vi "Read Joystick.vi"(8 "Joystick Deadbanded Value (default of 0.1)":dbl, 11 "Joystick L 1 DevRef":T1) -> (1 "Joystick L 2 X Axis":dbl, 2 "Joystick L 1 Y Axis":dbl, 3 "Joystick L 1 X Axis":dbl)   [LabVIEW 2014]
uses:
  <vilib>/Rock Robotics/WPI/Joystick/WPI_JoystickDevRef.ctl
  <vilib>/Rock Robotics/WPI/Joystick/WPI_JoystickDeviceEnum.ctl
  Global Variables.vi
  <vilib>/Rock Robotics/WPI/Joystick/WPI_JoystickGetSetRefNum.vi
  <vilib>/Utility/file.llb/Write To Spreadsheet File (DBL).vi
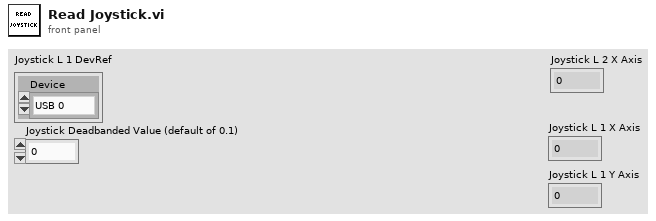
[diagram p1: front panel]
types:
  T1 = typedef "WPI_JoystickDevRef.ctl" = cluster{"Device":T2}
  T2 = typedef "WPI_JoystickDeviceEnum.ctl" = enum16{"USB 0", "USB 1", "USB 2", "USB 3", "USB 4", "USB 5"}
  T3 = cluster{"Buttons[0]":bool, "Buttons[1]":bool, "Buttons[2]":bool, "Buttons[3]":bool, "Buttons[4]":bool, "Buttons[5]":bool, "Buttons[6]":bool, "Buttons[7]":bool, "Buttons[8]":bool}
  T4 = cluster{"Axes[0]":dbl, "Axes[1]":dbl, "Axes[2]":dbl, "Axes[3]":dbl, "Axes[4]":dbl, "Axes[5]":dbl, "Axes[6]":dbl, "Axes[7]":dbl, "Axes[8]":dbl}
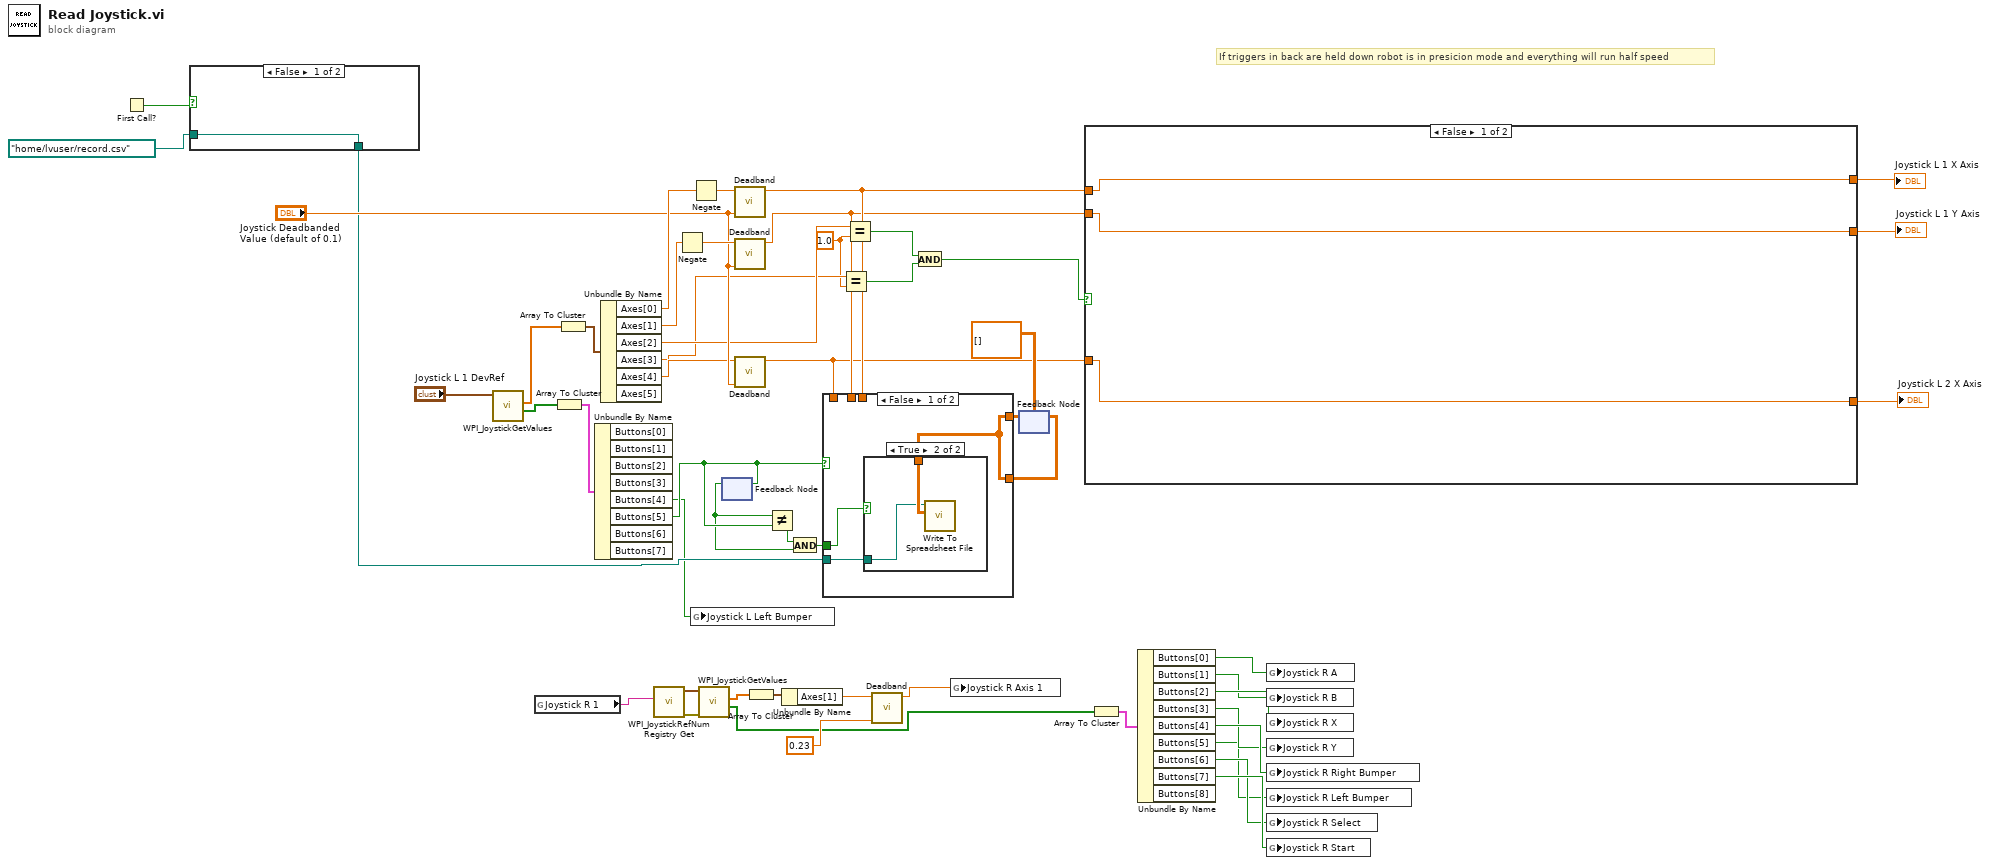
[diagram p0: block diagram]
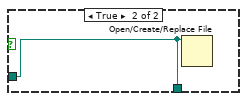
[diagram p2: hidden frame]
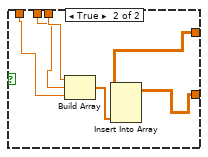
[diagram p4: hidden frame]
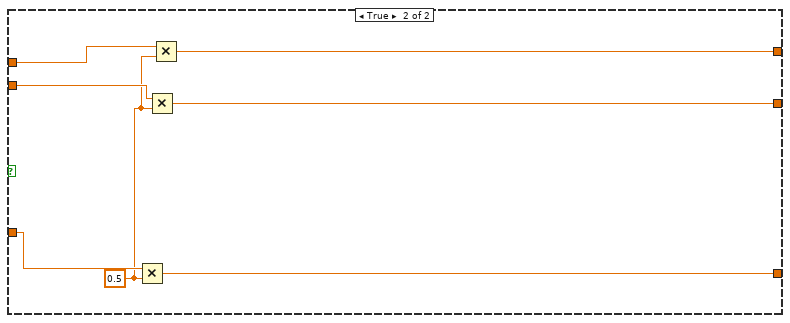
[diagram p5: hidden frame]
diagram:
  w22 = 1.0 ("y")
  # "If triggers in back are held down robot is in presicion mode and everything will run half speed"
  n1 = First Call?() -> (First Call?: T/F=w5:bool)
  n2 = case shown="False" w5 {
    tunnel: [w53 w54] -> w4
    tunnel: path "/home/lvuser/record.csv" ("file path (use dialog)") -> [w53 w54]
    frame False {
    }
    frame True {
      n3 = Open/Create/Replace File(file path (use dialog)=w54) -> ()  [unwired: 5 in, 3 out]
    }
  }
  n4 = call <vilib>:"WPI_JoystickGetValues.vi"("JoystickDevRef"="Joystick L 1 DevRef") -> ("Buttons"=w49:bool[], "Axes"=w51:dbl[])  [unwired: 6 in, 3 out]
  n5 = global read "Global Variables.vi" "Joystick R 1"() -> (w40:string)
  n6 = Array To Cluster(array=w49) -> (cluster=w48:T3)
  n7 = Array To Cluster(array=w51) -> (cluster=w50:T4)
  n8 = Unbundle By Name(w48) -> ("Buttons[4]"=w1:bool, "Buttons[5]"=w8:bool)  [unwired: 6 out]
  n9 = Unbundle By Name(w50) -> ("Axes[0]"=w47:dbl, "Axes[1]"=w44:dbl, "Axes[2]"=w24:dbl, "Axes[3]"=w23:dbl, "Axes[4]"=w25:dbl)  [unwired: 1 out]
  n10 = call <vilib>:"WPI_JoystickRefNum Registry Get.vi"("refnum name"=w40) -> ("error out"=w39:errorcluster, "JoystickDevRef"=w38:T1)  [unwired: 9 in]
  n11 = Negate(x=w44) -> (-x=w45:dbl)
  n12 = Negate(x=w47) -> (-x=w46:dbl)
  n13 = global write "Global Variables.vi" "Joystick L Left Bumper"(w1) -> ()
  n14 = call <vilib>:"WPI_JoystickGetValues.vi"("error in (no error)"=w39, "JoystickDevRef"=w38) -> ("Buttons"=w27:bool[], "Axes"=w41:dbl[])  [unwired: 5 in, 3 out]
  n15 = feedback #1() -> (w7:bool)  [unwired: 1 in]
  n16 = feedback-in #1(w8) -> ()
  n17 = call "Deadband.vi"("Value to Deadband (default of 0.1)"="Joystick Deadbanded Value (default of 0.1)", "Value"=w46) -> ("Deadbanded Value"=w15:dbl)  [unwired: 9 in]
  n18 = call "Deadband.vi"("Value to Deadband (default of 0.1)"="Joystick Deadbanded Value (default of 0.1)", "Value"=w45) -> ("Deadbanded Value"=w11:dbl)  [unwired: 9 in]
  n19 = call "Deadband.vi"("Value to Deadband (default of 0.1)"="Joystick Deadbanded Value (default of 0.1)", "Value"=w25) -> ("Deadbanded Value"=w10:dbl)  [unwired: 9 in]
  n20 = Array To Cluster(array=w41) -> (cluster=w42:T4)
  n21 = Not Equal?(x=w7, y=w8) -> (x != y?=w9:bool)
  n22 = Unbundle By Name(w42) -> ("Axes[1]"=w36:dbl)
  n23 = And(x=w9, y=w7) -> (x .and. y?=w6:bool)
  n24 = Equal?(x=w23, y=w22) -> (x = y?=w20:bool)
  n25 = Equal?(x=w24, y=w22) -> (x = y?=w21:bool)
  n26 = call "Deadband.vi"("Value to Deadband (default of 0.1)"=0.23, "Value"=w36) -> ("Deadbanded Value"=w35:dbl)  [unwired: 9 in]
  n27 = And(x=w21, y=w20) -> (x .and. y?=w19:bool)
  n28 = global write "Global Variables.vi" "Joystick R Axis 1"(w35) -> ()
  n29 = feedback #2(dbl[][] []) -> (w13:dbl[][])
  n30 = case shown="False" w8 {
    tunnel: w15 -> [_ w63]
    tunnel: [w56 w65] -> w14
    tunnel: w13 -> [w56 w64]
    tunnel: w11 -> [_ w62]
    tunnel: w10 -> [_ w61]
    tunnel: w6 -> [w57 _]
    tunnel: w4 -> [w55 _]
    frame False {
      n31 = case shown="True" w57 {
        tunnel: w56 -> [_ w59]
        tunnel: w55 -> [_ w58]
        frame False {
        }
        frame True {
          n32 = call-poly <vilib>:"Write To Spreadsheet File.vi"("2D data"=w59, "file path (dialog if empty)"=w58) -> ()  [unwired: 6 in, 1 out]
        }
      }
    }
    frame True {
      n33 = Build Array(w63, w62, w61) -> (w60:dbl[])
      n34 = Insert Into Array(array=w64, new element=w60) -> (w65:dbl[][])  [unwired: 2 in]
    }
  }
  n35 = feedback-in #2(w14) -> ()
  n36 = case shown="False" w19 {
    tunnel: w10 -> [w66 w75]
    tunnel: w11 -> [w67 w74]
    tunnel: w15 -> [w68 w72]
    tunnel: [w68 w71] -> w18
    tunnel: [w67 w70] -> w17
    tunnel: [w66 w69] -> w16
    frame False {
    }
    frame True {
      w73 = 0.5 ("y")
      n37 = Multiply(x=w75, y=w73) -> (x*y=w69:dbl)
      n38 = Multiply(x=w74, y=w73) -> (x*y=w70:dbl)
      n39 = Multiply(x=w72, y=w73) -> (x*y=w71:dbl)
    }
  }
  "Joystick L 1 Y Axis" <- w17
  "Joystick L 1 X Axis" <- w18
  "Joystick L 2 X Axis" <- w16
  n40 = Array To Cluster(array=w27) -> (cluster=w28:T3)
  n41 = Unbundle By Name(w28) -> ("Buttons[0]"=w26:bool, "Buttons[1]"=w29:bool, "Buttons[2]"=w30:bool, "Buttons[3]"=w31:bool, "Buttons[4]"=w32:bool, "Buttons[5]"=w2:bool, "Buttons[6]"=w33:bool, "Buttons[7]"=w34:bool)  [unwired: 1 out]
  n42 = global write "Global Variables.vi" "Joystick R A"(w26) -> ()
  n43 = global write "Global Variables.vi" "Joystick R B"(w29) -> ()
  n44 = global write "Global Variables.vi" "Joystick R X"(w30) -> ()
  n45 = global write "Global Variables.vi" "Joystick R Y"(w31) -> ()
  n46 = global write "Global Variables.vi" "Joystick R Right Bumper"(w32) -> ()
  n47 = global write "Global Variables.vi" "Joystick R Left Bumper"(w2) -> ()
  n48 = global write "Global Variables.vi" "Joystick R Select"(w33) -> ()
  n49 = global write "Global Variables.vi" "Joystick R Start"(w34) -> ()
